vi "Autonomous Independent.vi"   [LabVIEW 2013]
doc: "This VI is called when autonomous begins, and will automatically be terminated when autonomous ends. You can carry out timed or sensor driven robot movement independently without needing to return to the caller."
uses:
  <vilib>/Rock Robotics/WPI/SafetyOutput/WPI_SafetyOutputConfigMenu.ctl
  Robot Global Data.vi
  <vilib>/Rock Robotics/WPI/Solenoid/Deprecated/WPI_SolenoidSetBool.vi
  <vilib>/Rock Robotics/WPI/Joystick/WPI_JoystickGetSetRefNum.vi
  <vilib>/Rock Robotics/WPI/RobotDrive/WPI_RobotDriveGetSetRefNum.vi
panel:
  # "Be sure to right-click and choose Data Operations>>Make Current Value default if you want to save the array values with the VI"
types:
  T1 = typedef "WPI_SafetyOutputConfigMenu.ctl" = enum16{"Enable", "Disable"}
  T2 = typedef "WPI_JoystickDevRef.ctl" = cluster{"Device":T3}
  T3 = typedef "WPI_JoystickDeviceEnum.ctl" = enum16{"USB 1", "USB 2", "USB 3", "USB 4", "Kinect 1", "Kinect 2"}
  T4 = cluster{"axis 1 (x)":dbl, "axis 2 (y)":dbl, "axis 3 (throttle)":dbl, "axis 4":dbl, "axis 5":dbl, "axis 6":dbl}
  T5 = typedef "WPI_SolenoidDevRef.ctl" = cluster{"DevStatus":errorcluster, "Solenoid Module":T6, "Forward Solenoid Channel":T7, "Reverse Solenoid Channel":T7}
  T6 = typedef "FPGA_TypedefSolenoidModule.ctl" = enum16{"Solenoid Module 1", "Solenoid Module 2"}
  T7 = typedef "WPI_SolenoidChannel.ctl" = enum8{"Solenoid 1", "Solenoid 2", "Solenoid 3", "Solenoid 4", "Solenoid 5", "Solenoid 6", "Solenoid 7", "Solenoid 8", "Invalid"}
  T8 = typedef "WPI_RobotDriveDevRef.ctl" = cluster{"DevStatus":errorcluster, "Motors[]":T9[], "Square Inputs":bool, "Max Output":dbl, "Isochronous":bool}
  T9 = typedef "WPI_MotorControlDeviceRef.ctl" = cluster{"DeviceStatus":errorcluster, "Type":enum16{"PWM", "CAN"}, "PWM":cluster{"Digital Module":T10, "PWM Channel":T11, "DeadBand":T12}, "CAN":cluster{"Device Number":u8, "Control Mode":T13, "Semaphore":T14, "Max Vout":dbl}, "Invert":bool, "TransformRef":T15, "InvTransformRef":T15}
  T10 = typedef "FPGA_TypedefDigitalModule.ctl" = enum16{"Digital Module 1", "Digital Module 2"}
  T11 = typedef "FPGA_DIOPWMChannel.ctl" = enum8{"PWM 1", "PWM 2", "PWM 3", "PWM 4", "PWM 5", "PWM 6", "PWM 7", "PWM 8", "PWM 9", "PWM 10", "Invalid"}
  T12 = typedef "WPI_PWMDeadband.ctl" = cluster{"Name":string, "maxPositivePwm":i32, "minPositivePwm":i32, "centerPwm":i32, "maxNegativePwm":i32, "minNegativePwm":i32, "angularRange":u16}
  T13 = typedef "WPI_CANJaguar_ControlMode.ctl" = enum8{"Percent VBus", "Current", "Speed", "Position", "Voltage"}
  T14 = typedef "Semaphore RefNum" = refnum<k1>
  T15 = typedef "WPI_PWMTransform_ConPane.ctl" = refnum<vi>
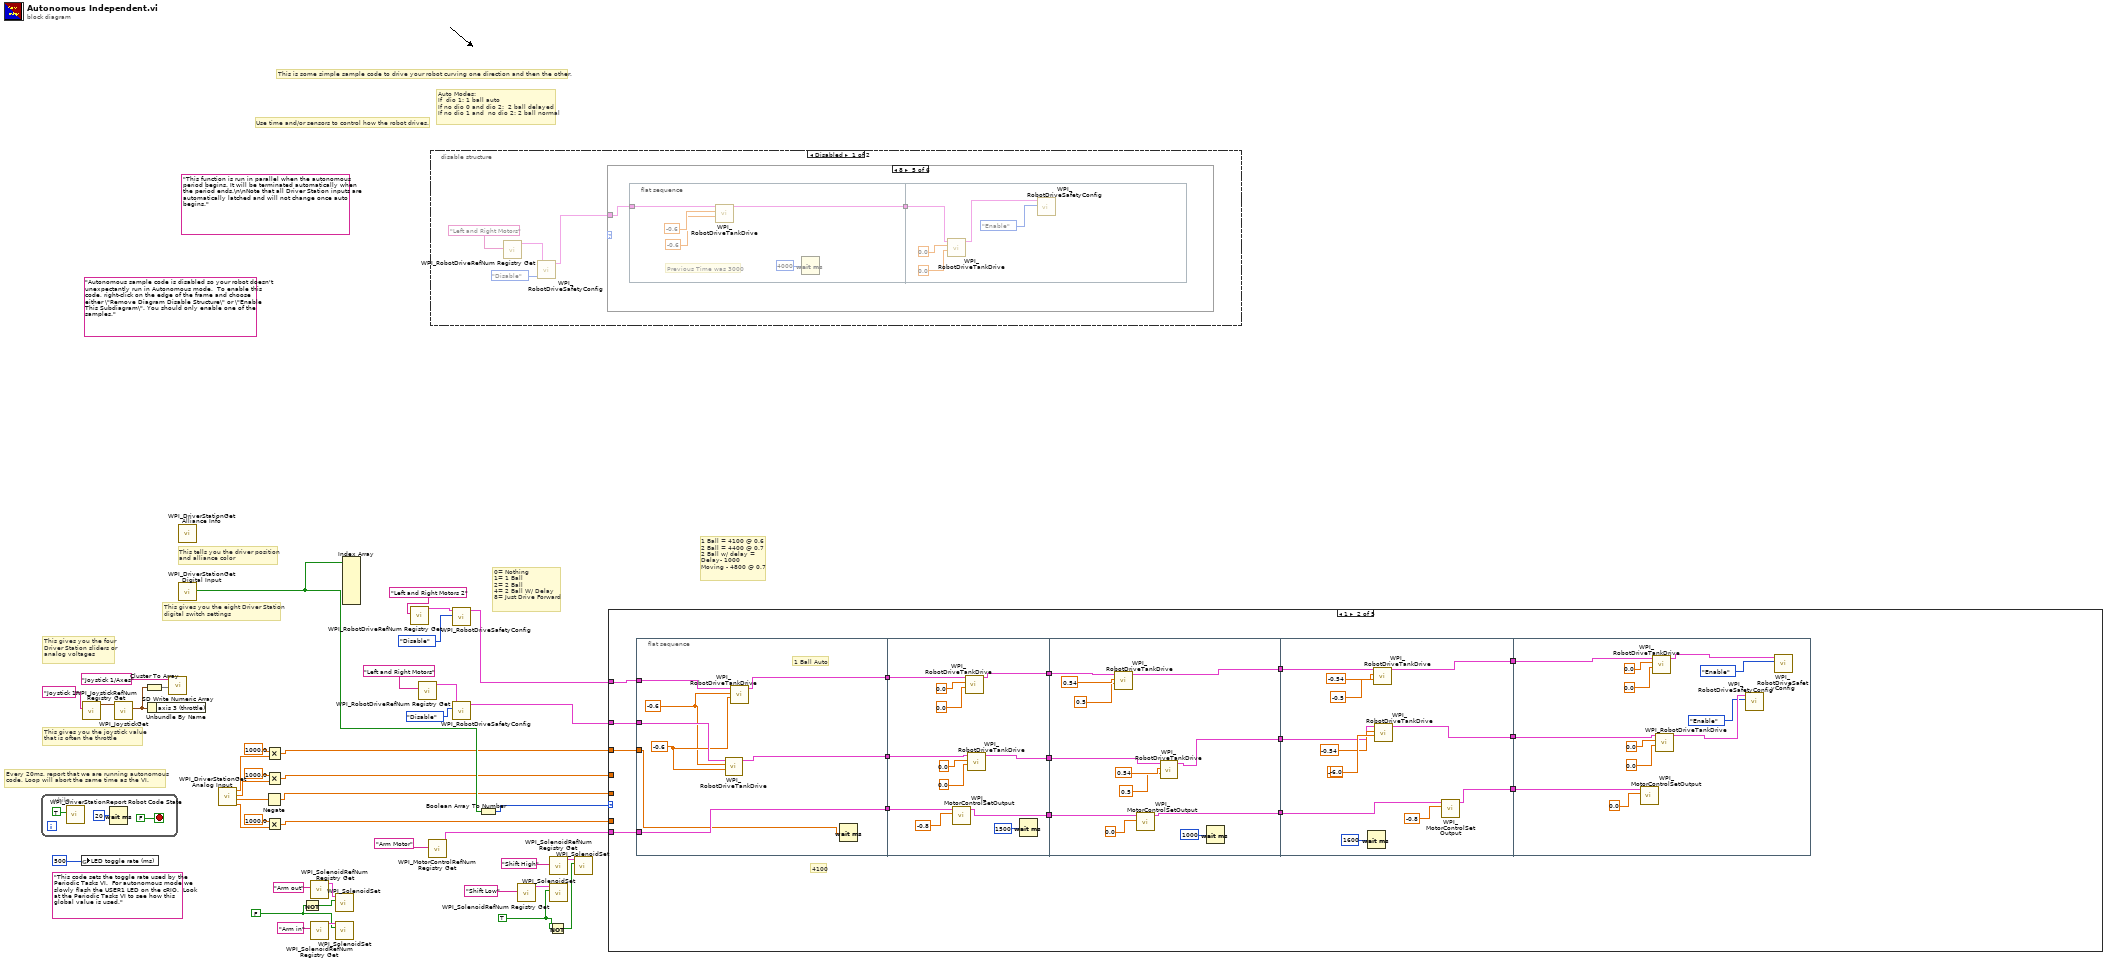
[diagram p0: block diagram]
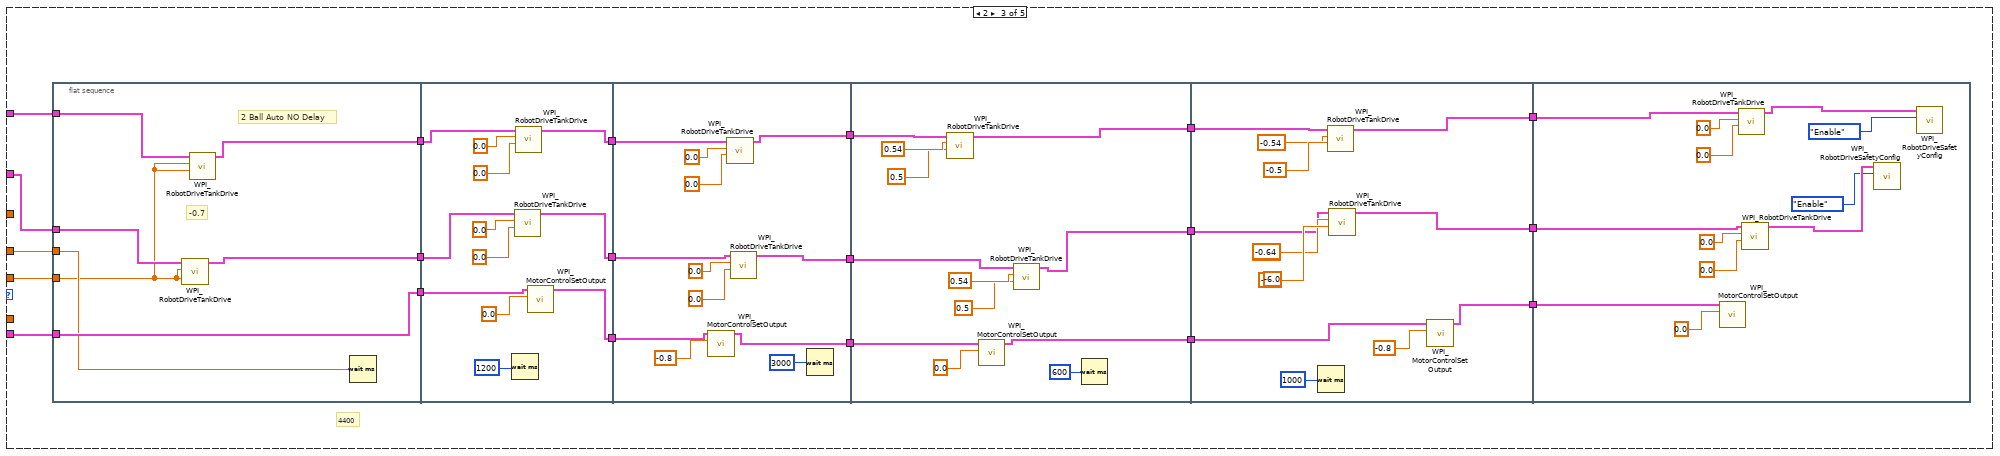
[diagram p3: hidden frame]
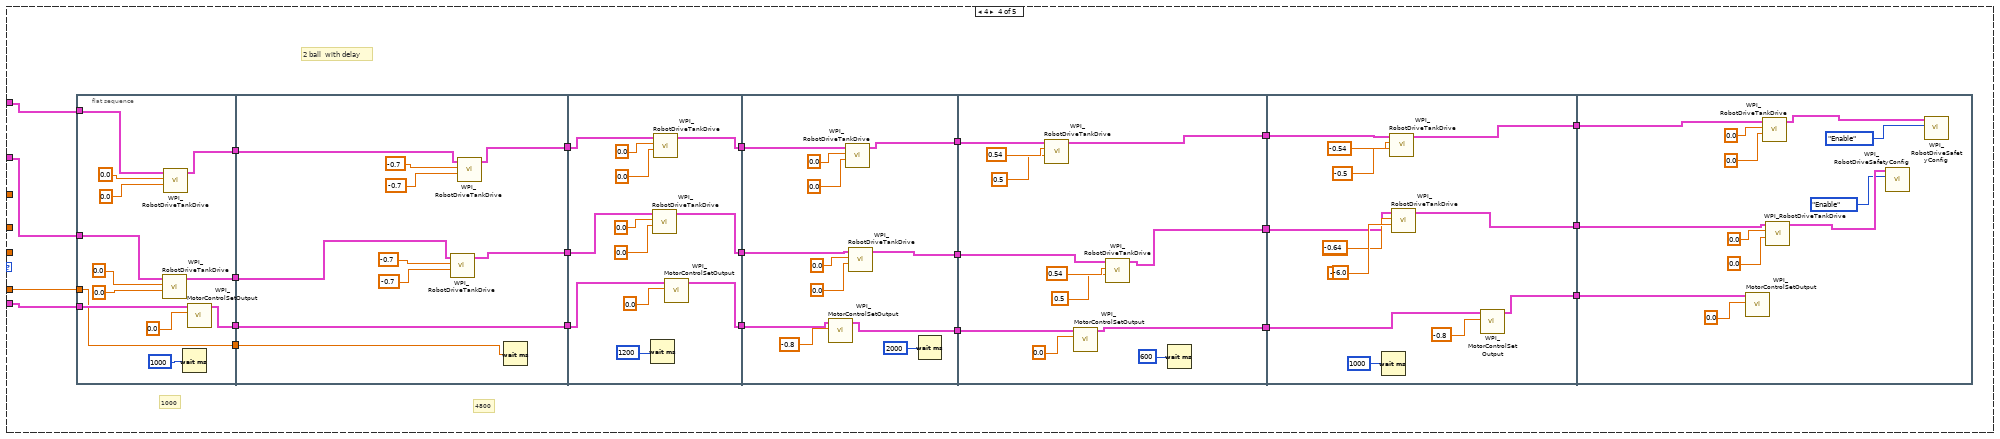
[diagram p4: hidden frame]
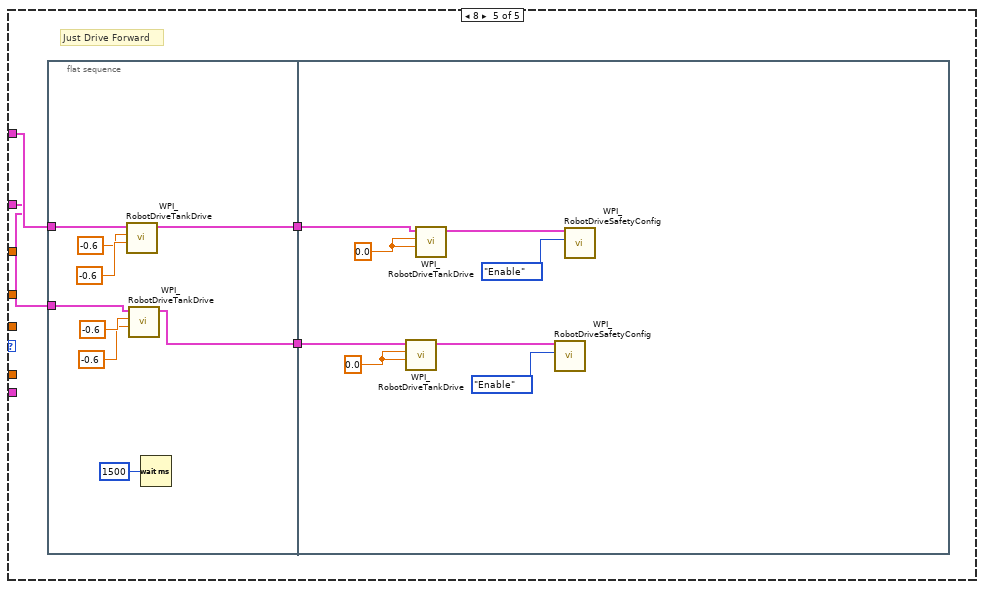
[diagram p5: hidden frame]
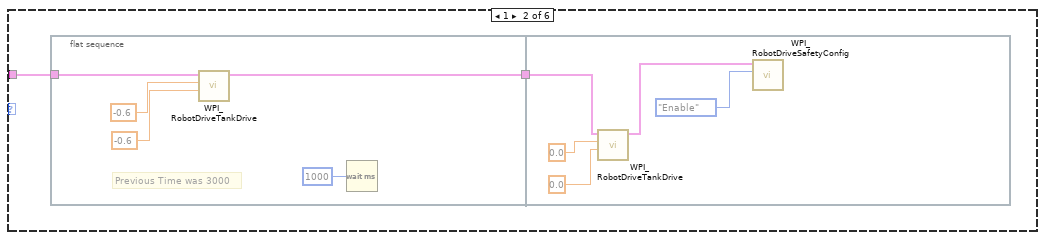
[diagram p7: hidden frame]
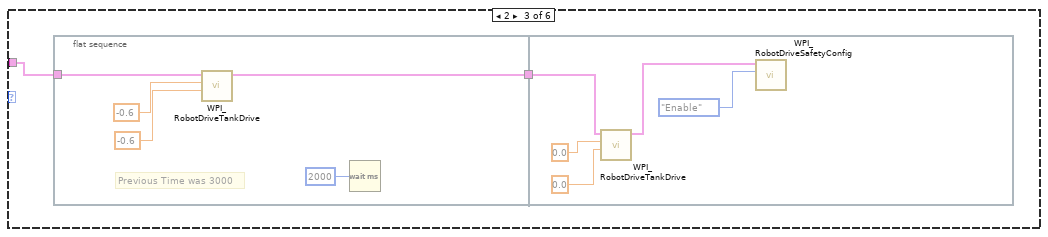
[diagram p8: hidden frame]
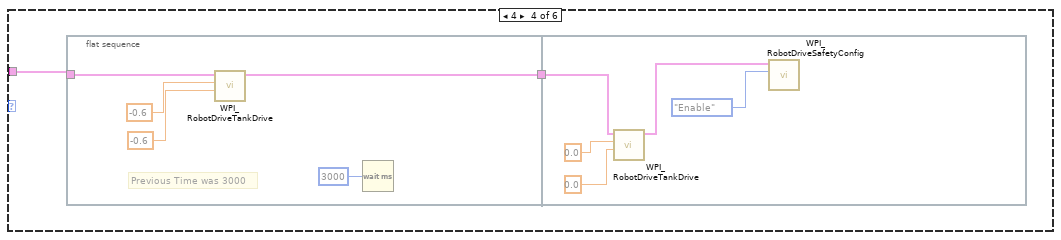
[diagram p9: hidden frame]
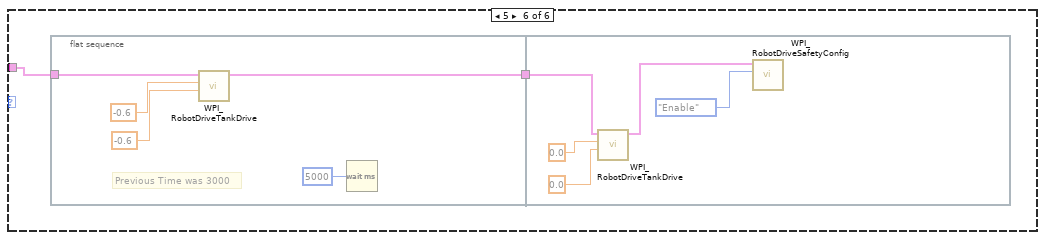
[diagram p10: hidden frame]
diagram:
  w1 = FALSE
  w26 = TRUE
  (unwired) "This code sets the toggle rate used by the Periodic Tasks VI.  For autonomous mode we slowly flash the USER1 LED on the cRIO.  Look at the Periodic Tasks VI to see how this global value is used."
  (unwired) "Autonomous sample code is disabled so your robot doesn't unexpectantly run in Autonomous mode.  To enable this code, right-click on the edge of the frame and choose either \"Remove Diagram Disable Structure\" or \"Enable This Subdiagram\". You should only enable one of the samples."
  (unwired) "This function is run in parallel when the autonomous period begins. It will be terminated automatically when the period ends.\n\nNote that all Driver Station inputs are automatically latched and will not change once auto begins."
  # "1 Ball = 4100 @ 0.6\n2 Ball = 4400 @ 0.7\n2 Ball w/ delay =\nDelay- 1000\nMoving - 4800 @ 0.7"
  # "0= Nothing\n1= 1 Ball\n2= 2 Ball\n4= 2 Ball W/ Delay\n8= Just Drive Forward"
  # "Auto Modes:\nIf  dio 1: 1 ball auto\nIf no dio 0 and dio 2:  2 ball delayed\nIf no dio 1 and  no dio 2: 2 ball normal"
  # "This is some simple sample code to drive your robot curving one direction and then the other."
  # "Every 20ms, report that we are running autonomous\ncode. Loop will abort the same time as the VI."
  # "This gives you the joystick value\nthat is often the throttle"
  # "Use time and/or sensors to control how the robot drives."
  # "This tells you the driver position\nand alliance color"
  # "This gives you the eight Driver Station\ndigital switch settings"
  # "This gives you the four\nDriver Station sliders or\nanalog voltages"
  n1 = while {
    stop <- FALSE stop-if-true
    n2 = call <vilib>:"WPI_DriverStationReport Robot Code State.vi"("Autonomous"=TRUE) -> ()  [unwired: 10 in, 1 out]
    n3 = Wait (ms)(milliseconds to wait=u32 20) -> ()  [unwired: 1 out]
  }
  n4 = global write "Robot Global Data.vi" "LED toggle rate (ms)"(u32 500 ("LED ms toggle rate")) -> ()
  n5 = call <vilib>:"WPI_JoystickRefNum Registry Get.vi"("refnum name"="Joystick 1") -> ("JoystickDevRef"=w40:T2)  [unwired: 1 in, 9 out]
  n6 = call <vilib>:"WPI_JoystickGet.vi"("JoystickDevRef"=w40) -> ("Axes"=w37:T4)  [unwired: 1 in, 5 out]
  n7 = Cluster To Array(cluster=w37) -> (array=w38:dbl[])
  n8 = Unbundle By Name(w37) -> ()  [unwired: 1 out]
  n9 = call <vilib>:"SD Write Numeric Array.vi"("Numeric Array"=w38, "Name"="Joystick 1/Axes") -> ()  [unwired: 8 in, 2 out]
  n10 = call <vilib>:"WPI_DriverStationGet Alliance Info.vi"() -> ()  [unwired: 12 out]
  n11 = call <vilib>:"WPI_DriverStationGet Digital Input.vi"() -> ("Driver Station Digital Input (1-8)"=w19:bool[])  [unwired: 11 out]
  n12 = call <vilib>:"WPI_DriverStationGet Analog Input.vi"() -> ("Analog 4 (V)"=w8:dbl, "Analog 3 (V)"=w9:dbl, "Analog 2 (V)"=w14:dbl, "Analog 1 (V)"=w15:dbl)  [unwired: 8 out]
  n13 = Negate(x=w9) -> (-x=w7:dbl)
  n14 = Multiply(x=1000.0, y=w15) -> (x*y=w12:dbl)
  n15 = Multiply(x=1000.0, y=w14) -> (x*y=w11:dbl)
  n16 = Multiply(x=1000.0, y=w8) -> (x*y=w10:dbl)
  n17 = Not(x=w1) -> (.not. x?=w2:bool)
  n18 = call <vilib>:"WPI_SolenoidRefNum Registry Get.vi"("refnum name"="Arm out") -> ("SolenoidDevRef"=w5:T5)  [unwired: 9 in, 1 out]
  n19 = call <vilib>:"WPI_SolenoidRefNum Registry Get.vi"("refnum name"="Arm in") -> ("SolenoidDevRef"=w4:T5)  [unwired: 9 in, 1 out]
  n20 = call-poly <vilib>:"WPI_SolenoidSet.vi"("Value"=w2, "SolenoidDevRef"=w5) -> ()  [unwired: 8 in, 2 out]
  n21 = call-poly <vilib>:"WPI_SolenoidSet.vi"("Value"=w1, "SolenoidDevRef"=w4) -> ()  [unwired: 8 in, 2 out]
  n22 = Index Array(array=w19) -> ()  [unwired: 8 in, 8 out]
  n23 = call <vilib>:"WPI_RobotDriveRefNum Registry Get.vi"("refnum name"="Left and Right Motors 2") -> ("RobotDriveDevRef"=w24:T8)  [unwired: 1 in, 9 out]
  n24 = call <vilib>:"WPI_RobotDriveRefNum Registry Get.vi"("refnum name"="Left and Right Motors") -> ("RobotDriveDevRef"=w33:T8)  [unwired: 1 in, 9 out]
  n25 = call <vilib>:"WPI_MotorControlRefNum Registry Get.vi"("refnum name"="Arm Motor") -> ("MotorControlDevRef"=w18:T9)  [unwired: 9 in, 1 out]
  n26 = disable-structure shown="Disabled" {
    frame Disabled {
      n27 = call <vilib>:"WPI_RobotDriveRefNum Registry Get.vi"("refnum name"="Left and Right Motors") -> ("RobotDriveDevRef"=w47:T8)  [unwired: 1 in, 9 out]
      n28 = call <vilib>:"WPI_RobotDriveSafetyConfig.vi"("mode"=WPI_SafetyOutputConfigMenu."Disable", "RobotDriveDevRef"=w47) -> ("RobotDriveDevRef"=w45:T8)  [unwired: 8 in, 1 out]
      n29 = case shown="8" {
        selector: _ -> [_ _ _ _ _ _]
        tunnel: w45 -> [_ w50 w61 w73 w85 w97]
        frame 0, Default {
        }
        frame 1 {
          n30 = flat-sequence {
            tunnel: w50 -> [w52]
            tunnel: [w51] -> w49
            tunnel: w49 -> [w57]
            frame #0 {
              # "Previous Time was 3000"
              n31 = call <vilib>:"WPI_RobotDriveTankDrive.vi"("Right axis value"=-0.6 ("X axis value"), "Left axis value"=-0.6 ("X axis value"), "RobotDriveDevRef"=w52) -> ("RobotDriveDevRef"=w51:T8)  [unwired: 6 in, 2 out]
              n32 = Wait (ms)(milliseconds to wait=u32 1000) -> ()  [unwired: 1 out]
            }
            frame #1 {
              n33 = call <vilib>:"WPI_RobotDriveTankDrive.vi"("Right axis value"=0.0 ("X axis value"), "Left axis value"=0.0 ("X axis value"), "RobotDriveDevRef"=w57) -> ("RobotDriveDevRef"=w56:T8)  [unwired: 6 in, 2 out]
              n34 = call <vilib>:"WPI_RobotDriveSafetyConfig.vi"("mode"=WPI_SafetyOutputConfigMenu."Enable", "RobotDriveDevRef"=w56) -> ()  [unwired: 8 in, 2 out]
            }
          }
        }
        frame 2 {
          n35 = flat-sequence {
            tunnel: w61 -> [w64]
            tunnel: [w63] -> w62
            tunnel: w62 -> [w69]
            frame #0 {
              # "Previous Time was 3000"
              n36 = call <vilib>:"WPI_RobotDriveTankDrive.vi"("Right axis value"=-0.6 ("X axis value"), "Left axis value"=-0.6 ("X axis value"), "RobotDriveDevRef"=w64) -> ("RobotDriveDevRef"=w63:T8)  [unwired: 6 in, 2 out]
              n37 = Wait (ms)(milliseconds to wait=u32 2000) -> ()  [unwired: 1 out]
            }
            frame #1 {
              n38 = call <vilib>:"WPI_RobotDriveTankDrive.vi"("Right axis value"=0.0 ("X axis value"), "Left axis value"=0.0 ("X axis value"), "RobotDriveDevRef"=w69) -> ("RobotDriveDevRef"=w68:T8)  [unwired: 6 in, 2 out]
              n39 = call <vilib>:"WPI_RobotDriveSafetyConfig.vi"("mode"=WPI_SafetyOutputConfigMenu."Enable", "RobotDriveDevRef"=w68) -> ()  [unwired: 8 in, 2 out]
            }
          }
        }
        frame 4 {
          n40 = flat-sequence {
            tunnel: w73 -> [w76]
            tunnel: [w75] -> w74
            tunnel: w74 -> [w81]
            frame #0 {
              # "Previous Time was 3000"
              n41 = call <vilib>:"WPI_RobotDriveTankDrive.vi"("Right axis value"=-0.6 ("X axis value"), "Left axis value"=-0.6 ("X axis value"), "RobotDriveDevRef"=w76) -> ("RobotDriveDevRef"=w75:T8)  [unwired: 6 in, 2 out]
              n42 = Wait (ms)(milliseconds to wait=u32 3000) -> ()  [unwired: 1 out]
            }
            frame #1 {
              n43 = call <vilib>:"WPI_RobotDriveTankDrive.vi"("Right axis value"=0.0 ("X axis value"), "Left axis value"=0.0 ("X axis value"), "RobotDriveDevRef"=w81) -> ("RobotDriveDevRef"=w80:T8)  [unwired: 6 in, 2 out]
              n44 = call <vilib>:"WPI_RobotDriveSafetyConfig.vi"("mode"=WPI_SafetyOutputConfigMenu."Enable", "RobotDriveDevRef"=w80) -> ()  [unwired: 8 in, 2 out]
            }
          }
        }
        frame 8 {
          n45 = flat-sequence {
            tunnel: w85 -> [w88]
            tunnel: [w87] -> w86
            tunnel: w86 -> [w93]
            frame #0 {
              # "Previous Time was 3000"
              n46 = call <vilib>:"WPI_RobotDriveTankDrive.vi"("Right axis value"=-0.6 ("X axis value"), "Left axis value"=-0.6 ("X axis value"), "RobotDriveDevRef"=w88) -> ("RobotDriveDevRef"=w87:T8)  [unwired: 6 in, 2 out]
              n47 = Wait (ms)(milliseconds to wait=u32 4000) -> ()  [unwired: 1 out]
            }
            frame #1 {
              n48 = call <vilib>:"WPI_RobotDriveTankDrive.vi"("Right axis value"=0.0 ("X axis value"), "Left axis value"=0.0 ("X axis value"), "RobotDriveDevRef"=w93) -> ("RobotDriveDevRef"=w92:T8)  [unwired: 6 in, 2 out]
              n49 = call <vilib>:"WPI_RobotDriveSafetyConfig.vi"("mode"=WPI_SafetyOutputConfigMenu."Enable", "RobotDriveDevRef"=w92) -> ()  [unwired: 8 in, 2 out]
            }
          }
        }
        frame 5 {
          n50 = flat-sequence {
            tunnel: w97 -> [w100]
            tunnel: [w99] -> w98
            tunnel: w98 -> [w105]
            frame #0 {
              # "Previous Time was 3000"
              n51 = call <vilib>:"WPI_RobotDriveTankDrive.vi"("Right axis value"=-0.6 ("X axis value"), "Left axis value"=-0.6 ("X axis value"), "RobotDriveDevRef"=w100) -> ("RobotDriveDevRef"=w99:T8)  [unwired: 6 in, 2 out]
              n52 = Wait (ms)(milliseconds to wait=u32 5000) -> ()  [unwired: 1 out]
            }
            frame #1 {
              n53 = call <vilib>:"WPI_RobotDriveTankDrive.vi"("Right axis value"=0.0 ("X axis value"), "Left axis value"=0.0 ("X axis value"), "RobotDriveDevRef"=w105) -> ("RobotDriveDevRef"=w104:T8)  [unwired: 6 in, 2 out]
              n54 = call <vilib>:"WPI_RobotDriveSafetyConfig.vi"("mode"=WPI_SafetyOutputConfigMenu."Enable", "RobotDriveDevRef"=w104) -> ()  [unwired: 8 in, 2 out]
            }
          }
        }
      }
    }
    frame Enabled {
    }
  }
  n55 = call <vilib>:"WPI_RobotDriveSafetyConfig.vi"("mode"=WPI_SafetyOutputConfigMenu."Disable", "RobotDriveDevRef"=w24) -> ("RobotDriveDevRef"=w22:T8)  [unwired: 8 in, 1 out]
  n56 = call <vilib>:"WPI_RobotDriveSafetyConfig.vi"("mode"=WPI_SafetyOutputConfigMenu."Disable", "RobotDriveDevRef"=w33) -> ("RobotDriveDevRef"=w21:T8)  [unwired: 8 in, 1 out]
  n57 = Boolean Array To Number(Boolean array=w19) -> (number=w20:u32)
  n58 = call <vilib>:"WPI_SolenoidRefNum Registry Get.vi"("refnum name"="Shift Low") -> ("SolenoidDevRef"=w30:T5)  [unwired: 9 in, 1 out]
  n59 = Not(x=w26) -> (.not. x?=w27:bool)
  n60 = call <vilib>:"WPI_SolenoidRefNum Registry Get.vi"("refnum name"="Shift High") -> ("SolenoidDevRef"=w29:T5)  [unwired: 9 in, 1 out]
  n61 = call-poly <vilib>:"WPI_SolenoidSet.vi"("Value"=w26, "SolenoidDevRef"=w30) -> ()  [unwired: 8 in, 2 out]
  n62 = call-poly <vilib>:"WPI_SolenoidSet.vi"("Value"=w27, "SolenoidDevRef"=w29) -> ()  [unwired: 8 in, 2 out]
  n63 = case shown="1" w20 {
    tunnel: w22 -> [_ w113 w186 w272 w375]
    tunnel: w21 -> [_ w112 w185 w271 w374]
    tunnel: w18 -> [_ w110 w183 w270 _]
    tunnel: w12 -> [_ w109 _ _ _]
    tunnel: w11 -> [_ _ w182 _ _]
    tunnel: w10 -> [_ _ _ w268 _]
    tunnel: w7 -> [_ _ w181 _ _]
    frame 0, Default {
      # "Do Nothing at all"
    }
    frame 1 {
      # "4100"
      n64 = flat-sequence {
        tunnel: [w132] -> w124
        tunnel: [w131] -> w123
        tunnel: w113 -> [w130]
        tunnel: w112 -> [w129]
        tunnel: [w128] -> w111
        tunnel: w110 -> [w128]
        tunnel: w109 -> [w125]
        tunnel: [w142] -> w122
        tunnel: w124 -> [w141]
        tunnel: [w140] -> w121
        tunnel: w123 -> [w135]
        tunnel: [w134] -> w120
        tunnel: w111 -> [w133]
        tunnel: w122 -> [w155]
        tunnel: w121 -> [w154]
        tunnel: w120 -> [w150]
        tunnel: [w148] -> w119
        tunnel: [w147] -> w118
        tunnel: [w146] -> w117
        tunnel: w119 -> [w166]
        tunnel: w118 -> [w163]
        tunnel: w117 -> [w161]
        tunnel: [w159] -> w116
        tunnel: [w158] -> w115
        tunnel: [w157] -> w114
        tunnel: w116 -> [w175]
        tunnel: w115 -> [w171]
        tunnel: w114 -> [w170]
        frame #0 {
          w127 = -0.6 ("X axis value")
          w126 = -0.6 ("X axis value")
          # "1 Ball Auto"
          n65 = call <vilib>:"WPI_RobotDriveTankDrive.vi"("Right axis value"=w127, "Left axis value"=w126, "RobotDriveDevRef"=w129) -> ("RobotDriveDevRef"=w132:T8)  [unwired: 6 in, 2 out]
          n66 = call <vilib>:"WPI_RobotDriveTankDrive.vi"("Right axis value"=w127, "Left axis value"=w126, "RobotDriveDevRef"=w130) -> ("RobotDriveDevRef"=w131:T8)  [unwired: 6 in, 2 out]
          n67 = Wait (ms)(milliseconds to wait=w125) -> ()  [unwired: 1 out]
        }
        frame #1 {
          n68 = call <vilib>:"WPI_MotorControlSetOutput.vi"("Output"=-0.8, "MotorControlDevRef"=w133) -> ("MotorControlDevRef"=w142:T9)  [unwired: 7 in, 2 out]
          n69 = call <vilib>:"WPI_RobotDriveTankDrive.vi"("Right axis value"=0.0 ("X axis value"), "Left axis value"=0.0 ("X axis value"), "RobotDriveDevRef"=w135) -> ("RobotDriveDevRef"=w134:T8)  [unwired: 6 in, 2 out]
          n70 = call <vilib>:"WPI_RobotDriveTankDrive.vi"("Right axis value"=0.0 ("X axis value"), "Left axis value"=0.0 ("X axis value"), "RobotDriveDevRef"=w141) -> ("RobotDriveDevRef"=w140:T8)  [unwired: 6 in, 2 out]
          n71 = Wait (ms)(milliseconds to wait=u32 1500) -> ()  [unwired: 1 out]
        }
        frame #2 {
          n72 = call <vilib>:"WPI_RobotDriveTankDrive.vi"("Right axis value"=0.5 ("X axis value"), "Left axis value"=0.54 ("X axis value"), "RobotDriveDevRef"=w150) -> ("RobotDriveDevRef"=w148:T8)  [unwired: 6 in, 2 out]
          n73 = call <vilib>:"WPI_MotorControlSetOutput.vi"("Output"=0.0, "MotorControlDevRef"=w155) -> ("MotorControlDevRef"=w146:T9)  [unwired: 7 in, 2 out]
          n74 = call <vilib>:"WPI_RobotDriveTankDrive.vi"("Right axis value"=0.5 ("X axis value"), "Left axis value"=0.54 ("X axis value"), "RobotDriveDevRef"=w154) -> ("RobotDriveDevRef"=w147:T8)  [unwired: 6 in, 2 out]
          n75 = Wait (ms)(milliseconds to wait=u32 1000) -> ()  [unwired: 1 out]
        }
        frame #3 {
          (unwired) -6.0 ("X axis value")
          n76 = Wait (ms)(milliseconds to wait=u32 1600) -> ()  [unwired: 1 out]
          n77 = call <vilib>:"WPI_RobotDriveTankDrive.vi"("Right axis value"=-0.5 ("X axis value"), "Left axis value"=-0.54 ("X axis value"), "RobotDriveDevRef"=w166) -> ("RobotDriveDevRef"=w158:T8)  [unwired: 6 in, 2 out]
          n78 = call <vilib>:"WPI_RobotDriveTankDrive.vi"("Right axis value"=-0.5 ("X axis value"), "Left axis value"=-0.54 ("X axis value"), "RobotDriveDevRef"=w163) -> ("RobotDriveDevRef"=w159:T8)  [unwired: 6 in, 2 out]
          n79 = call <vilib>:"WPI_MotorControlSetOutput.vi"("Output"=-0.8, "MotorControlDevRef"=w161) -> ("MotorControlDevRef"=w157:T9)  [unwired: 7 in, 2 out]
        }
        frame #4 {
          n80 = call <vilib>:"WPI_MotorControlSetOutput.vi"("Output"=0.0, "MotorControlDevRef"=w170) -> ()  [unwired: 7 in, 3 out]
          n81 = call <vilib>:"WPI_RobotDriveTankDrive.vi"("Right axis value"=0.0 ("X axis value"), "Left axis value"=0.0 ("X axis value"), "RobotDriveDevRef"=w171) -> ("RobotDriveDevRef"=w172:T8)  [unwired: 6 in, 2 out]
          n82 = call <vilib>:"WPI_RobotDriveTankDrive.vi"("Right axis value"=0.0 ("X axis value"), "Left axis value"=0.0 ("X axis value"), "RobotDriveDevRef"=w175) -> ("RobotDriveDevRef"=w174:T8)  [unwired: 6 in, 2 out]
          n83 = call <vilib>:"WPI_RobotDriveSafetyConfig.vi"("mode"=WPI_SafetyOutputConfigMenu."Enable", "RobotDriveDevRef"=w174) -> ()  [unwired: 8 in, 2 out]
          n84 = call <vilib>:"WPI_RobotDriveSafetyConfig.vi"("mode"=WPI_SafetyOutputConfigMenu."Enable", "RobotDriveDevRef"=w172) -> ()  [unwired: 8 in, 2 out]
        }
      }
    }
    frame 2 {
      # "4400"
      n85 = flat-sequence {
        tunnel: [w207] -> w200
        tunnel: [w206] -> w199
        tunnel: w186 -> [w205]
        tunnel: w185 -> [w204]
        tunnel: [w203] -> w184
        tunnel: w183 -> [w203]
        tunnel: w182 -> [w202]
        tunnel: w181 -> [w201]
        tunnel: w200 -> [w213]
        tunnel: w199 -> [w212]
        tunnel: [w211] -> w198
        tunnel: [w210] -> w197
        tunnel: [w209] -> w196
        tunnel: w184 -> [w208]
        tunnel: [w228] -> w195
        tunnel: [w226] -> w194
        tunnel: [w220] -> w193
        tunnel: w198 -> [w221]
        tunnel: w197 -> [w227]
        tunnel: w196 -> [w231]
        tunnel: w195 -> [w242]
        tunnel: w194 -> [w241]
        tunnel: w193 -> [w236]
        tunnel: [w234] -> w192
        tunnel: [w233] -> w191
        tunnel: [w232] -> w190
        tunnel: w192 -> [w253]
        tunnel: w191 -> [w250]
        tunnel: w190 -> [w248]
        tunnel: [w246] -> w189
        tunnel: [w245] -> w188
        tunnel: [w244] -> w187
        tunnel: w189 -> [w262]
        tunnel: w188 -> [w258]
        tunnel: w187 -> [w257]
        frame #0 {
          # "-0.7"
          # "2 Ball Auto NO Delay"
          n86 = call <vilib>:"WPI_RobotDriveTankDrive.vi"("Right axis value"=w201, "Left axis value"=w201, "RobotDriveDevRef"=w204) -> ("RobotDriveDevRef"=w207:T8)  [unwired: 6 in, 2 out]
          n87 = call <vilib>:"WPI_RobotDriveTankDrive.vi"("Right axis value"=w201, "Left axis value"=w201, "RobotDriveDevRef"=w205) -> ("RobotDriveDevRef"=w206:T8)  [unwired: 6 in, 2 out]
          n88 = Wait (ms)(milliseconds to wait=w202) -> ()  [unwired: 1 out]
        }
        frame #1 {
          n89 = Wait (ms)(milliseconds to wait=u32 1200) -> ()  [unwired: 1 out]
          n90 = call <vilib>:"WPI_RobotDriveTankDrive.vi"("Right axis value"=0.0 ("X axis value"), "Left axis value"=0.0 ("X axis value"), "RobotDriveDevRef"=w213) -> ("RobotDriveDevRef"=w210:T8)  [unwired: 6 in, 2 out]
          n91 = call <vilib>:"WPI_RobotDriveTankDrive.vi"("Right axis value"=0.0 ("X axis value"), "Left axis value"=0.0 ("X axis value"), "RobotDriveDevRef"=w212) -> ("RobotDriveDevRef"=w211:T8)  [unwired: 6 in, 2 out]
          n92 = call <vilib>:"WPI_MotorControlSetOutput.vi"("Output"=0.0, "MotorControlDevRef"=w208) -> ("MotorControlDevRef"=w209:T9)  [unwired: 7 in, 2 out]
        }
        frame #2 {
          n93 = call <vilib>:"WPI_MotorControlSetOutput.vi"("Output"=-0.8, "MotorControlDevRef"=w231) -> ("MotorControlDevRef"=w228:T9)  [unwired: 7 in, 2 out]
          n94 = call <vilib>:"WPI_RobotDriveTankDrive.vi"("Right axis value"=0.0 ("X axis value"), "Left axis value"=0.0 ("X axis value"), "RobotDriveDevRef"=w221) -> ("RobotDriveDevRef"=w220:T8)  [unwired: 6 in, 2 out]
          n95 = call <vilib>:"WPI_RobotDriveTankDrive.vi"("Right axis value"=0.0 ("X axis value"), "Left axis value"=0.0 ("X axis value"), "RobotDriveDevRef"=w227) -> ("RobotDriveDevRef"=w226:T8)  [unwired: 6 in, 2 out]
          n96 = Wait (ms)(milliseconds to wait=u32 3000) -> ()  [unwired: 1 out]
        }
        frame #3 {
          n97 = call <vilib>:"WPI_RobotDriveTankDrive.vi"("Right axis value"=0.5 ("X axis value"), "Left axis value"=0.54 ("X axis value"), "RobotDriveDevRef"=w236) -> ("RobotDriveDevRef"=w234:T8)  [unwired: 6 in, 2 out]
          n98 = call <vilib>:"WPI_MotorControlSetOutput.vi"("Output"=0.0, "MotorControlDevRef"=w242) -> ("MotorControlDevRef"=w232:T9)  [unwired: 7 in, 2 out]
          n99 = call <vilib>:"WPI_RobotDriveTankDrive.vi"("Right axis value"=0.5 ("X axis value"), "Left axis value"=0.54 ("X axis value"), "RobotDriveDevRef"=w241) -> ("RobotDriveDevRef"=w233:T8)  [unwired: 6 in, 2 out]
          n100 = Wait (ms)(milliseconds to wait=u32 600) -> ()  [unwired: 1 out]
        }
        frame #4 {
          (unwired) -0.64 ("X axis value")
          (unwired) -6.0 ("X axis value")
          n101 = Wait (ms)(milliseconds to wait=u32 1000) -> ()  [unwired: 1 out]
          n102 = call <vilib>:"WPI_RobotDriveTankDrive.vi"("Right axis value"=-0.5 ("X axis value"), "Left axis value"=-0.54 ("X axis value"), "RobotDriveDevRef"=w253) -> ("RobotDriveDevRef"=w245:T8)  [unwired: 6 in, 2 out]
          n103 = call <vilib>:"WPI_RobotDriveTankDrive.vi"("Right axis value"=-0.5 ("X axis value"), "Left axis value"=-0.54 ("X axis value"), "RobotDriveDevRef"=w250) -> ("RobotDriveDevRef"=w246:T8)  [unwired: 6 in, 2 out]
          n104 = call <vilib>:"WPI_MotorControlSetOutput.vi"("Output"=-0.8, "MotorControlDevRef"=w248) -> ("MotorControlDevRef"=w244:T9)  [unwired: 7 in, 2 out]
        }
        frame #5 {
          n105 = call <vilib>:"WPI_MotorControlSetOutput.vi"("Output"=0.0, "MotorControlDevRef"=w257) -> ()  [unwired: 7 in, 3 out]
          n106 = call <vilib>:"WPI_RobotDriveTankDrive.vi"("Right axis value"=0.0 ("X axis value"), "Left axis value"=0.0 ("X axis value"), "RobotDriveDevRef"=w258) -> ("RobotDriveDevRef"=w259:T8)  [unwired: 6 in, 2 out]
          n107 = call <vilib>:"WPI_RobotDriveTankDrive.vi"("Right axis value"=0.0 ("X axis value"), "Left axis value"=0.0 ("X axis value"), "RobotDriveDevRef"=w262) -> ("RobotDriveDevRef"=w261:T8)  [unwired: 6 in, 2 out]
          n108 = call <vilib>:"WPI_RobotDriveSafetyConfig.vi"("mode"=WPI_SafetyOutputConfigMenu."Enable", "RobotDriveDevRef"=w261) -> ()  [unwired: 8 in, 2 out]
          n109 = call <vilib>:"WPI_RobotDriveSafetyConfig.vi"("mode"=WPI_SafetyOutputConfigMenu."Enable", "RobotDriveDevRef"=w259) -> ()  [unwired: 8 in, 2 out]
        }
      }
    }
    frame 4 {
      # "4800"
      # "1000"
      # "2 ball  with delay"
      n110 = flat-sequence {
        tunnel: [w298] -> w290
        tunnel: [w297] -> w289
        tunnel: [w296] -> w288
        tunnel: w272 -> [w294]
        tunnel: w271 -> [w293]
        tunnel: w270 -> [w292]
        tunnel: [w291] -> w269
        tunnel: w268 -> [w291]
        tunnel: [w313] -> w287
        tunnel: [w312] -> w286
        tunnel: [w307] -> w285
        tunnel: w290 -> [w313]
        tunnel: w289 -> [w306]
        tunnel: w288 -> [w305]
        tunnel: w269 -> [w304]
        tunnel: w287 -> [w319]
        tunnel: w286 -> [w318]
        tunnel: w285 -> [w317]
        tunnel: [w316] -> w284
        tunnel: [w315] -> w283
        tunnel: [w314] -> w282
        tunnel: [w334] -> w281
        tunnel: [w332] -> w280
        tunnel: [w326] -> w279
        tunnel: w284 -> [w327]
        tunnel: w283 -> [w333]
        tunnel: w282 -> [w337]
        tunnel: w281 -> [w348]
        tunnel: w280 -> [w347]
        tunnel: w279 -> [w342]
        tunnel: [w340] -> w278
        tunnel: [w339] -> w277
        tunnel: [w338] -> w276
        tunnel: w278 -> [w359]
        tunnel: w277 -> [w356]
        tunnel: w276 -> [w354]
        tunnel: [w352] -> w275
        tunnel: [w351] -> w274
        tunnel: [w350] -> w273
        tunnel: w275 -> [w368]
        tunnel: w274 -> [w364]
        tunnel: w273 -> [w363]
        frame #0 {
          n111 = call <vilib>:"WPI_RobotDriveTankDrive.vi"("Right axis value"=0.0 ("X axis value"), "Left axis value"=0.0 ("X axis value"), "RobotDriveDevRef"=w293) -> ("RobotDriveDevRef"=w297:T8)  [unwired: 6 in, 2 out]
          n112 = call <vilib>:"WPI_RobotDriveTankDrive.vi"("Right axis value"=0.0 ("X axis value"), "Left axis value"=0.0 ("X axis value"), "RobotDriveDevRef"=w294) -> ("RobotDriveDevRef"=w296:T8)  [unwired: 6 in, 2 out]
          n113 = Wait (ms)(milliseconds to wait=u32 1000) -> ()  [unwired: 1 out]
          n114 = call <vilib>:"WPI_MotorControlSetOutput.vi"("Output"=0.0, "MotorControlDevRef"=w292) -> ("MotorControlDevRef"=w298:T9)  [unwired: 7 in, 2 out]
        }
        frame #1 {
          n115 = call <vilib>:"WPI_RobotDriveTankDrive.vi"("Right axis value"=-0.7 ("X axis value"), "Left axis value"=-0.7 ("X axis value"), "RobotDriveDevRef"=w306) -> ("RobotDriveDevRef"=w312:T8)  [unwired: 6 in, 2 out]
          n116 = call <vilib>:"WPI_RobotDriveTankDrive.vi"("Right axis value"=-0.7 ("X axis value"), "Left axis value"=-0.7 ("X axis value"), "RobotDriveDevRef"=w305) -> ("RobotDriveDevRef"=w307:T8)  [unwired: 6 in, 2 out]
          n117 = Wait (ms)(milliseconds to wait=w304) -> ()  [unwired: 1 out]
        }
        frame #2 {
          n118 = Wait (ms)(milliseconds to wait=u32 1200) -> ()  [unwired: 1 out]
          n119 = call <vilib>:"WPI_RobotDriveTankDrive.vi"("Right axis value"=0.0 ("X axis value"), "Left axis value"=0.0 ("X axis value"), "RobotDriveDevRef"=w318) -> ("RobotDriveDevRef"=w315:T8)  [unwired: 6 in, 2 out]
          n120 = call <vilib>:"WPI_RobotDriveTankDrive.vi"("Right axis value"=0.0 ("X axis value"), "Left axis value"=0.0 ("X axis value"), "RobotDriveDevRef"=w317) -> ("RobotDriveDevRef"=w316:T8)  [unwired: 6 in, 2 out]
          n121 = call <vilib>:"WPI_MotorControlSetOutput.vi"("Output"=0.0, "MotorControlDevRef"=w319) -> ("MotorControlDevRef"=w314:T9)  [unwired: 7 in, 2 out]
        }
        frame #3 {
          n122 = call <vilib>:"WPI_MotorControlSetOutput.vi"("Output"=-0.8, "MotorControlDevRef"=w337) -> ("MotorControlDevRef"=w334:T9)  [unwired: 7 in, 2 out]
          n123 = call <vilib>:"WPI_RobotDriveTankDrive.vi"("Right axis value"=0.0 ("X axis value"), "Left axis value"=0.0 ("X axis value"), "RobotDriveDevRef"=w327) -> ("RobotDriveDevRef"=w326:T8)  [unwired: 6 in, 2 out]
          n124 = call <vilib>:"WPI_RobotDriveTankDrive.vi"("Right axis value"=0.0 ("X axis value"), "Left axis value"=0.0 ("X axis value"), "RobotDriveDevRef"=w333) -> ("RobotDriveDevRef"=w332:T8)  [unwired: 6 in, 2 out]
          n125 = Wait (ms)(milliseconds to wait=u32 2000) -> ()  [unwired: 1 out]
        }
        frame #4 {
          n126 = call <vilib>:"WPI_RobotDriveTankDrive.vi"("Right axis value"=0.5 ("X axis value"), "Left axis value"=0.54 ("X axis value"), "RobotDriveDevRef"=w342) -> ("RobotDriveDevRef"=w340:T8)  [unwired: 6 in, 2 out]
          n127 = call <vilib>:"WPI_MotorControlSetOutput.vi"("Output"=0.0, "MotorControlDevRef"=w348) -> ("MotorControlDevRef"=w338:T9)  [unwired: 7 in, 2 out]
          n128 = call <vilib>:"WPI_RobotDriveTankDrive.vi"("Right axis value"=0.5 ("X axis value"), "Left axis value"=0.54 ("X axis value"), "RobotDriveDevRef"=w347) -> ("RobotDriveDevRef"=w339:T8)  [unwired: 6 in, 2 out]
          n129 = Wait (ms)(milliseconds to wait=u32 600) -> ()  [unwired: 1 out]
        }
        frame #5 {
          (unwired) -0.64 ("X axis value")
          (unwired) -6.0 ("X axis value")
          n130 = Wait (ms)(milliseconds to wait=u32 1000) -> ()  [unwired: 1 out]
          n131 = call <vilib>:"WPI_RobotDriveTankDrive.vi"("Right axis value"=-0.5 ("X axis value"), "Left axis value"=-0.54 ("X axis value"), "RobotDriveDevRef"=w359) -> ("RobotDriveDevRef"=w351:T8)  [unwired: 6 in, 2 out]
          n132 = call <vilib>:"WPI_RobotDriveTankDrive.vi"("Right axis value"=-0.5 ("X axis value"), "Left axis value"=-0.54 ("X axis value"), "RobotDriveDevRef"=w356) -> ("RobotDriveDevRef"=w352:T8)  [unwired: 6 in, 2 out]
          n133 = call <vilib>:"WPI_MotorControlSetOutput.vi"("Output"=-0.8, "MotorControlDevRef"=w354) -> ("MotorControlDevRef"=w350:T9)  [unwired: 7 in, 2 out]
        }
        frame #6 {
          n134 = call <vilib>:"WPI_MotorControlSetOutput.vi"("Output"=0.0, "MotorControlDevRef"=w363) -> ()  [unwired: 7 in, 3 out]
          n135 = call <vilib>:"WPI_RobotDriveTankDrive.vi"("Right axis value"=0.0 ("X axis value"), "Left axis value"=0.0 ("X axis value"), "RobotDriveDevRef"=w364) -> ("RobotDriveDevRef"=w365:T8)  [unwired: 6 in, 2 out]
          n136 = call <vilib>:"WPI_RobotDriveTankDrive.vi"("Right axis value"=0.0 ("X axis value"), "Left axis value"=0.0 ("X axis value"), "RobotDriveDevRef"=w368) -> ("RobotDriveDevRef"=w367:T8)  [unwired: 6 in, 2 out]
          n137 = call <vilib>:"WPI_RobotDriveSafetyConfig.vi"("mode"=WPI_SafetyOutputConfigMenu."Enable", "RobotDriveDevRef"=w367) -> ()  [unwired: 8 in, 2 out]
          n138 = call <vilib>:"WPI_RobotDriveSafetyConfig.vi"("mode"=WPI_SafetyOutputConfigMenu."Enable", "RobotDriveDevRef"=w365) -> ()  [unwired: 8 in, 2 out]
        }
      }
    }
    frame 8 {
      # "Just Drive Forward"
      n139 = flat-sequence {
        tunnel: [w385] -> w377
        tunnel: [w380] -> w376
        tunnel: w375 -> [w379]
        tunnel: w374 -> [w378]
        tunnel: w377 -> [w394]
        tunnel: w376 -> [w387]
        frame #0 {
          n140 = call <vilib>:"WPI_RobotDriveTankDrive.vi"("Right axis value"=-0.6, "Left axis value"=-0.6, "RobotDriveDevRef"=w379) -> ("RobotDriveDevRef"=w385:T8)  [unwired: 6 in, 2 out]
          n141 = call <vilib>:"WPI_RobotDriveTankDrive.vi"("Right axis value"=-0.6, "Left axis value"=-0.6, "RobotDriveDevRef"=w378) -> ("RobotDriveDevRef"=w380:T8)  [unwired: 6 in, 2 out]
          n142 = Wait (ms)(milliseconds to wait=u32 1500) -> ()  [unwired: 1 out]
        }
        frame #1 {
          w390 = 0.0 ("Left axis value")
          w391 = 0.0 ("Left axis value")
          n143 = call <vilib>:"WPI_RobotDriveTankDrive.vi"("Right axis value"=w390, "Left axis value"=w390, "RobotDriveDevRef"=w387) -> ("RobotDriveDevRef"=w388:T8)  [unwired: 6 in, 2 out]
          n144 = call <vilib>:"WPI_RobotDriveTankDrive.vi"("Right axis value"=w391, "Left axis value"=w391, "RobotDriveDevRef"=w394) -> ("RobotDriveDevRef"=w393:T8)  [unwired: 6 in, 2 out]
          n145 = call <vilib>:"WPI_RobotDriveSafetyConfig.vi"("mode"=WPI_SafetyOutputConfigMenu."Enable", "RobotDriveDevRef"=w388) -> ()  [unwired: 8 in, 2 out]
          n146 = call <vilib>:"WPI_RobotDriveSafetyConfig.vi"("mode"=WPI_SafetyOutputConfigMenu."Enable", "RobotDriveDevRef"=w393) -> ()  [unwired: 8 in, 2 out]
        }
      }
    }
  }
